vi "basic - IRIG Time Control.vi"() -> ()   [LabVIEW 2020]
uses:
  _polimorphicInstances/session/Fdx Create Session (Generic-Board).vi
  _polimorphicInstances/session/Fdx Close Session (Board).vi
  AIM664LV.lvlib
panel:
  out "current irig time":T1={"SignOut"=40, "DayOut"=1, "HourOut"=1, "MinOut"=28, "SecondOut"=39, "MilliSecOut"=539, "MicroSecOut"=300, "NanoSecOut"=0, "InfoOut"=0, "Mode"=3}
  in  "Board Number":u32
  # "ARINC 664 IRIG Time Query"
  # "Overview: Obtain the IRIG time from the board.\n\nRequirement: One AIM ARINC-664 board with installed AIM ARINC 664 BSP.\nRestrictions: None.\nInstruction:\n1. Select the Board ID (0 if you have only one board in your system).\n2. Run the VI.\n3. See the result in Current IRIG Time"
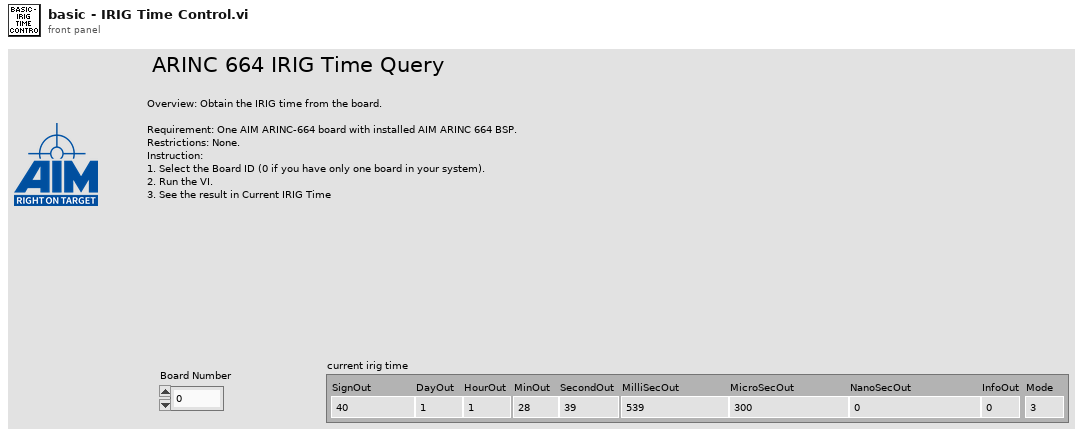
[diagram p1: front panel]
types:
  T1 = cluster{"SignOut":i32, "DayOut":u32, "HourOut":u32, "MinOut":u32, "SecondOut":u32, "MilliSecOut":u32, "MicroSecOut":u32, "NanoSecOut":u32, "InfoOut":u32, "Mode":u32}
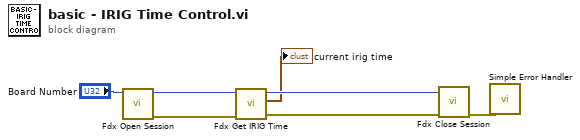
[diagram p0: block diagram]
diagram:
  n1 = call-poly "Fdx Open Session.vi"("board"="Board Number") -> ("error out"=w5:errorcluster, "InstrumentHandle_board out"=w6:u32)  [unwired: 8 in, 1 out]
  n2 = call "Fdx Get IRIG Time.vi"("error in (no error)"=w5, "InstrumentHandle_board in"=w6) -> ("error out"=w3:errorcluster, "Curent Irig Time"=→"current irig time":T1, "InstrumentHandle_board out"=w4:u32)  [unwired: 7 in]
  n3 = call-poly "Fdx Close Session.vi"("error in (no error)"=w3, "InstrumentHandle_board in"=w4) -> ("error out"=w1:errorcluster)  [unwired: 9 in]
  n4 = call <vilib>:"Simple Error Handler.vi"("error in (no error)"=w1) -> ()  [unwired: 4 in, 5 out]
